vi "DriveEnd.vi"() -> (0 "Error Out":errorcluster, 1 "Advance Trigger":bool)   [LabVIEW 2019]
doc: "Zeros out all drive-related joystick commands and stops the drive sequencer.\n\nParameters: None"
uses:
  dscommands.vi
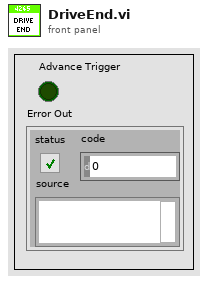
[diagram p1: front panel]
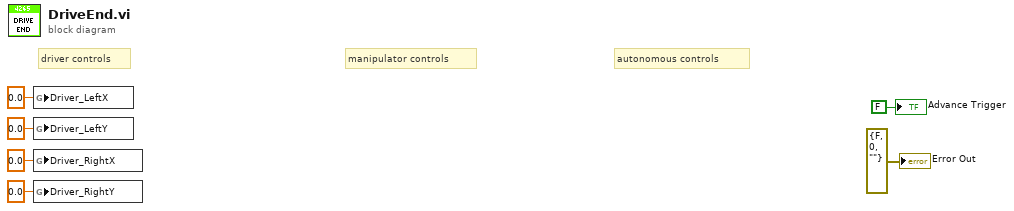
[diagram p0: block diagram]
diagram:
  # "manipulator controls"
  # "driver controls"
  # "autonomous controls"
  n1 = global write "dscommands.vi" "Driver_LeftX"(0.0 ("Driver_LeftX")) -> ()
  n2 = global write "dscommands.vi" "Driver_LeftY"(0.0 ("Driver_LeftY")) -> ()
  n3 = global write "dscommands.vi" "Driver_RightX"(0.0 ("Driver_RightX")) -> ()
  n4 = global write "dscommands.vi" "Driver_RightY"(0.0 ("Driver_RightY")) -> ()
  "Advance Trigger" <- FALSE ("Advance Trigger")
  "Error Out" <- errorcluster {"status"=FALSE, "code"=0, "source"=""} ("error constant")
